vi "Add ColumnHead Item by Text Width and TextAlign.vi"(7 "textAlign":i32(ring) items=["Left", "Right", "Center"], 8 "error in (no error)":errorcluster caption="错误输入（无错误）", 9 "width":i32, 10 "text":string, 11 "ListViewClass 输入":refnum<class "ListViewClass.lvclass"> caption="DNL_LabVIEW Object in") -> (0 "error out":errorcluster caption="错误输出", 3 "ListViewClass 输出":refnum<class "ListViewClass.lvclass"> caption="DNL_LabVIEW Object out")   [LabVIEW 2012, in "ListViewClass.lvclass"]
uses:
  ListViewClass.lvclass
  ListViewClass.lvclass/ListViewClass.ctl
  System.Windows.Forms
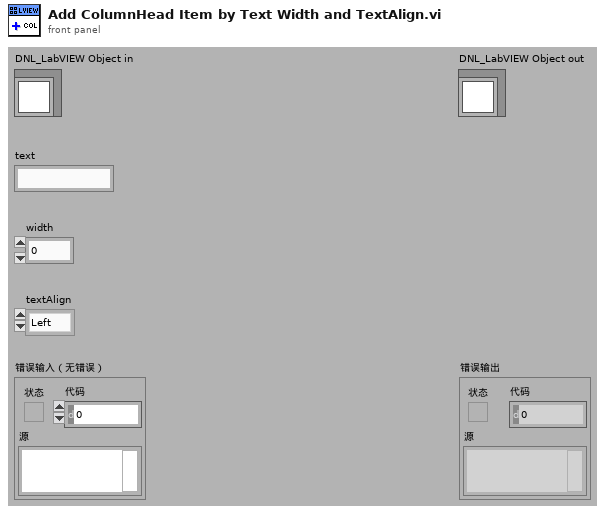
[diagram p1: front panel]
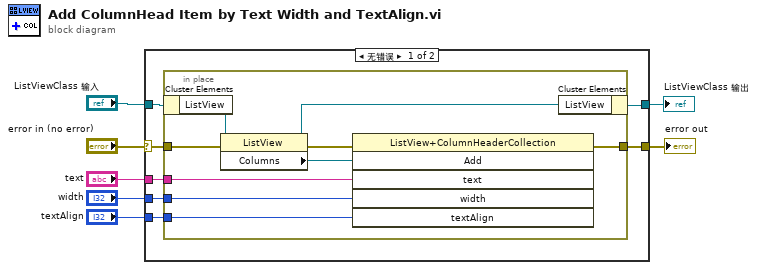
[diagram p0: block diagram]
diagram:
  n1 = case shown="无错误" "error in (no error)" {
    selector: "error in (no error)" -> [w9 w25]
    tunnel: [w8 w25] -> w6
    tunnel: [w13 w24] -> w4
    tunnel: "ListViewClass 输入" -> [w14 w24]
    tunnel: "text" -> [w12 _]
    tunnel: "width" -> [w11 _]
    tunnel: "textAlign" -> [w10 _]
    frame No Error {
      n2 = in-place {
        in-place-border: w12 -> [w20]
        in-place-border: w11 -> [w19]
        in-place-border: w10 -> [w18]
        in-place-border: w9 -> [w17]
        in-place-border: [w15] -> w8
        n3 = in-place-cluster #1(w14) -> ("ListView"=w23:refnum<k24>)
        n4 = property class="ListView"(reference=w23, error in=w17) -> (reference out=w21:refnum<k24>, error out=w16:errorcluster, "Columns"=w22:refnum<k24>)
        n5 = invoke class="ListView+ColumnHeaderCollection" method="Add"(reference=w22, error in=w16, "text"=w20, "width"=w19, "textAlign"=w18) -> (error out=w15:errorcluster)  [unwired: 1 in, 5 out]
        n6 = in-place-cluster #1("ListView"=w21) -> (w13:refnum<class "ListViewClass.lvclass">)
      }
    }
    frame Error {
    }
  }
  "error out" <- w6
  "ListViewClass 输出" <- w4
